vi "niDTS WLAN UTIL Gard Interval to RFSA Gard Interval.vi"(10 "Gard Interval":T1 caption="GI") -> (2 "CONFigure:RFSA:WLAN:MODulation:OFDM:GuardInterval":enum16{"LONG", "SHORt"}(ring))   [LabVIEW 2014, in "niDTS WLAN.lvlib"]
uses:
  niDTS WLAN.lvlib
  Includes/niDTS WLAN INC GI.ctl
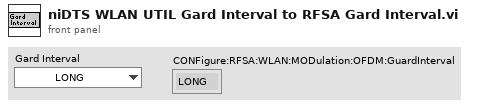
[diagram p1: front panel]
types:
  T1 = typedef "niDTS WLAN.lvlib/niDTS WLAN INC GI.ctl" = enum16{"LONG", "SHORT"}
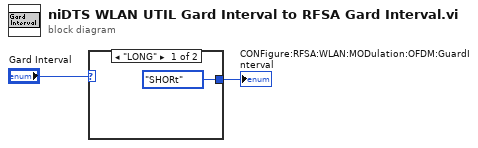
[diagram p0: block diagram]
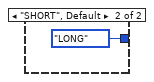
[diagram p2: hidden frame]
diagram:
  n1 = case shown="\"LONG\"" "Gard Interval" {
    tunnel: [enum16{"LONG", "SHORt"}."SHORt" ("CONFigure:RFSA:WLAN:MODulation:OFDM:GuardInterval") enum16{"LONG", "SHORt"}."LONG" ("CONFigure:RFSA:WLAN:MODulation:OFDM:GuardInterval")] -> w2
    frame "LONG" {
    }
    frame "SHORT", Default {
    }
  }
  "CONFigure:RFSA:WLAN:MODulation:OFDM:GuardInterval" <- w2
